vi "Update channel.vi"(8 "Error In":errorcluster, 9 "Value":dbl min=0.0 max=204.8000030517578 step=0.012500000186264515 format="%#_g V", 10 "Channel":u8 max=31 step=1, 11 "Arduino Port":refnum<visa-resource-name>) -> (0 "Error Out":errorcluster, 3 "Arduino Port out":refnum<visa-resource-name>)   [LabVIEW 2016]
doc: "Perform an update of the voltage output of the input channel of AD5535. The max speed of this operation is 1-2ms"
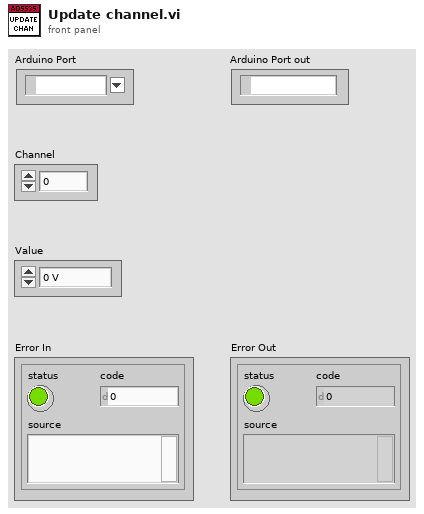
[diagram p1: front panel]
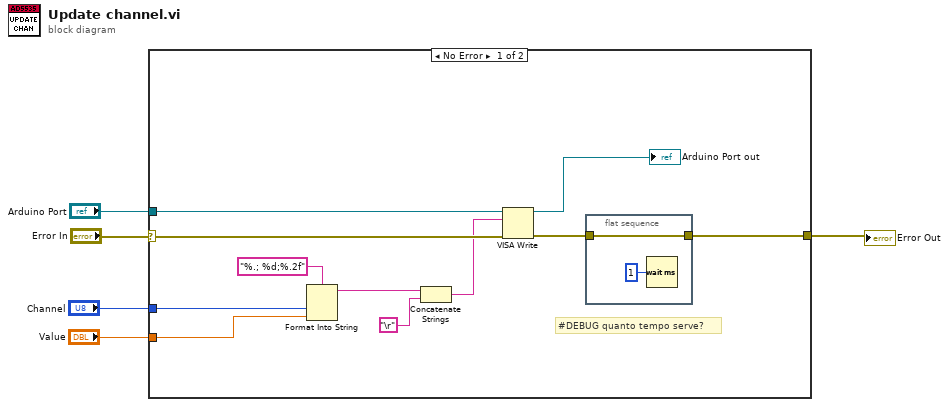
[diagram p0: block diagram]
diagram:
  n1 = case shown="No Error" "Error In" {
    selector: "Error In" -> [w15 w19]
    tunnel: [w6 w19] -> w4
    tunnel: "Arduino Port" -> [w16 _]
    tunnel: "Channel" -> [w13 _]
    tunnel: "Value" -> [w12 _]
    frame No Error {
      # "#DEBUG quanto tempo serve?"
      n2 = Format Into String(format string="%.; %d;%.2f", w13, w12) -> (resulting string=w10:string)  [unwired: 2 in, 1 out]
      n3 = Concatenate Strings(w10, "\r") -> (w8:string)
      n4 = VISA Write(VISA resource name=w16, write buffer=w8, error in (no error)=w15) -> (VISA resource name out=→"Arduino Port out":refnum<visa-resource-name>, error out=w7:errorcluster)  [unwired: 1 out]
      n5 = flat-sequence {
        tunnel: w7 -> [w18]
        tunnel: [w18] -> w6
        frame #0 {
          n6 = Wait (ms)(milliseconds to wait=u32 1) -> ()  [unwired: 1 out]
        }
      }
    }
    frame Error {
    }
  }
  "Error Out" <- w4
